vi "setDeviceParameters.vi"(8 "error in (no error)":errorcluster, 11 "RaspberryPi in":refnum<class "RaspberryPi.lvclass">) -> (0 "error out":errorcluster, 3 "RaspberryPi out":refnum<class "RaspberryPi.lvclass">)   [LabVIEW 2020, in "RaspberryPi.lvclass"]
uses:
  RaspberryPi.lvclass
  AutomatedController/AutomatedController.lvclass
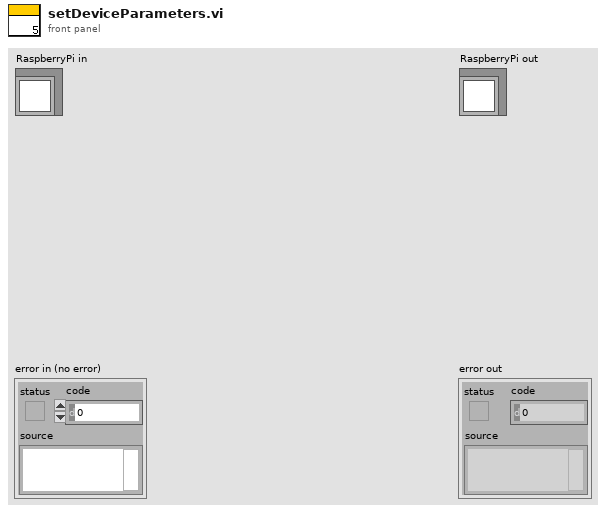
[diagram p1: front panel]
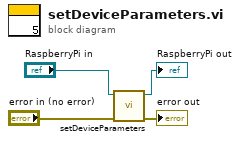
[diagram p0: block diagram]
diagram:
  n1 = call-parent "setDeviceParameters.vi"("error in (no error)"="error in (no error)", "AutomatedController in"="RaspberryPi in") -> ("error out"=→"error out":errorcluster, "AutomatedController out"=→"RaspberryPi out":refnum<class "RaspberryPi.lvclass">)  [unwired: 8 in]
